vi "oscilloscope.vi"() -> ()   [LabVIEW 2017]
uses:
  <vilib>/DAQmx/read.llb/DAQmx Read (Analog Wfm 1Chan NSamp).vi
  <vilib>/DAQmx/create/channels.llb/DAQmx Create Channel (AI-Voltage-Basic).vi
  <vilib>/DAQmx/configure/timing.llb/DAQmx Timing (Sample Clock).vi
  <vilib>/DAQmx/miscellaneous.llb/DAQmx Fill In Error Info.vi
  <vilib>/Waveform/WDTOps.llb/WDT Get XY Value DBL.vi
panel:
  in  "physical channels":tag="cDAQ9185-1D03A69Mod1/ai14"
  out "Waveform Graph":waveform(dbl)(graph)
  out "Numeric":dbl
  in  "Stop Button":bool
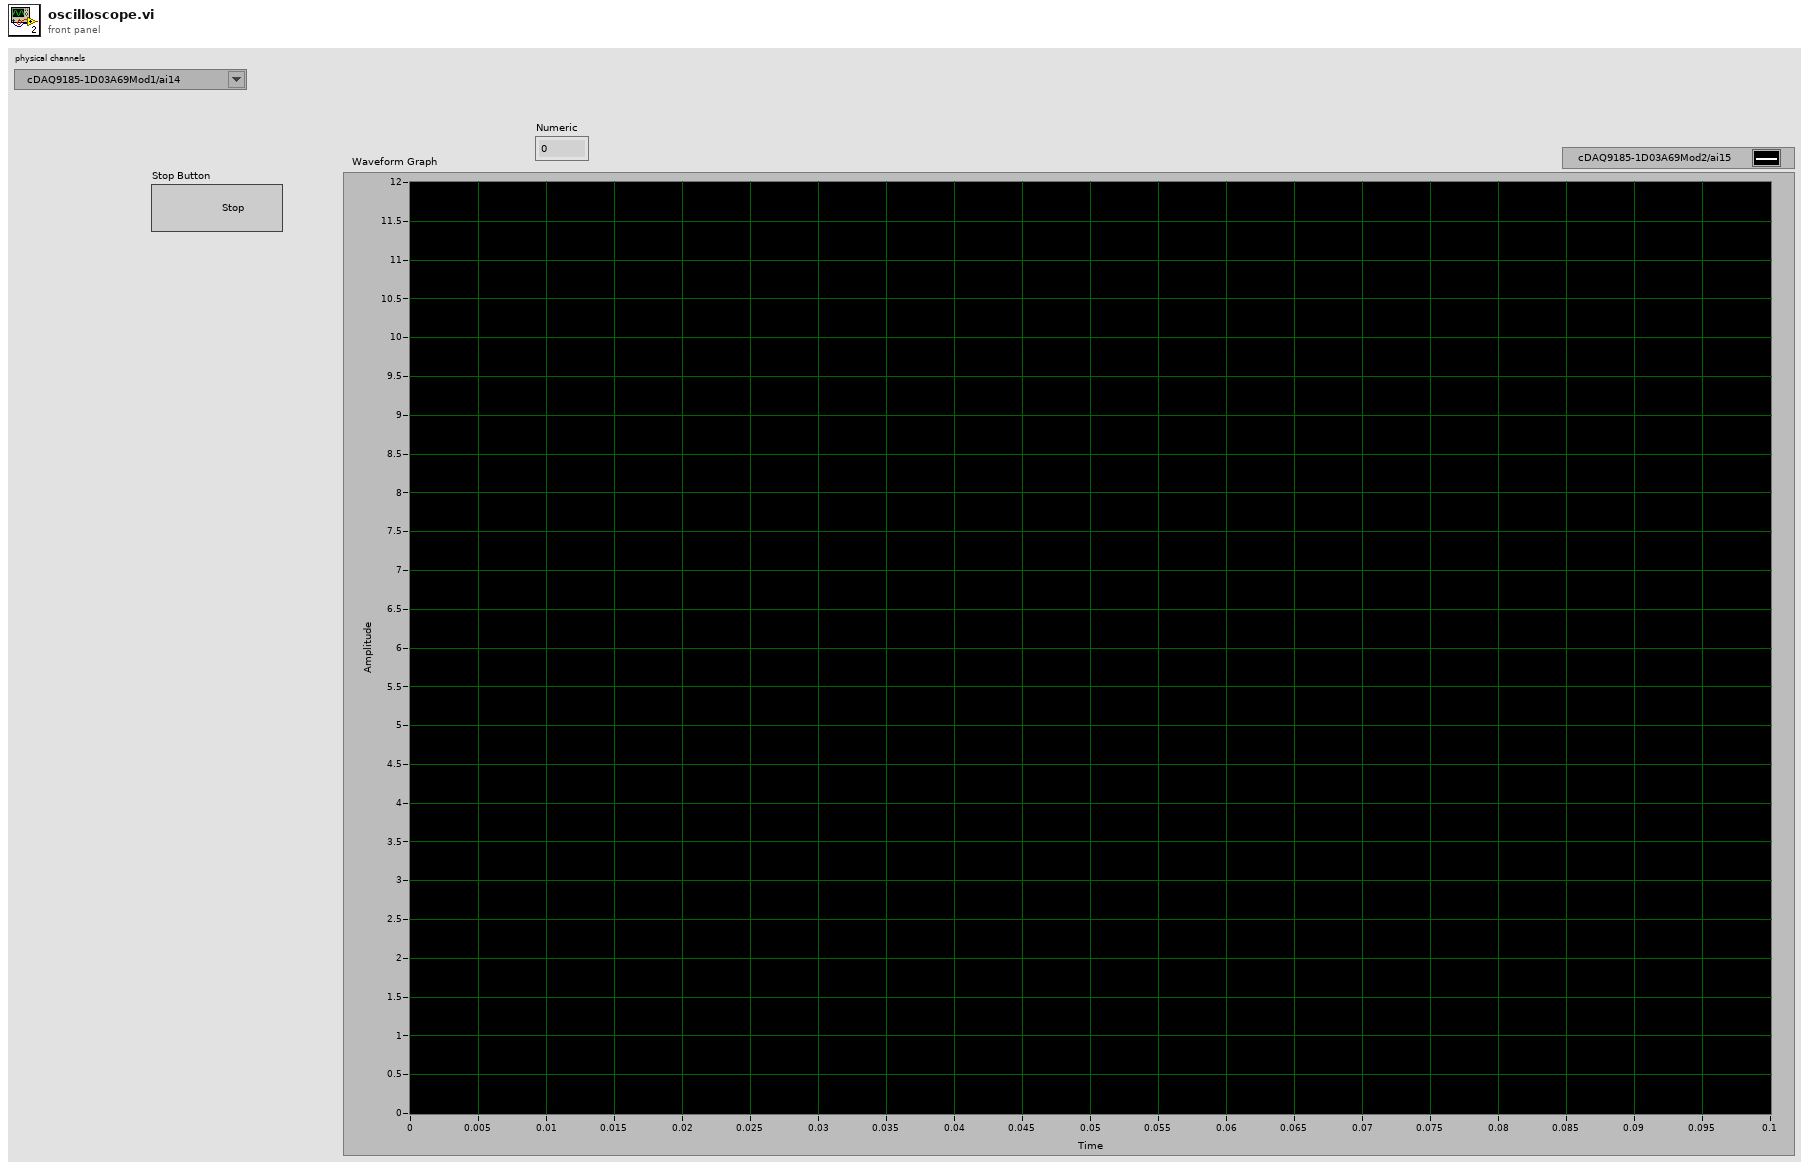
[diagram p1: front panel]
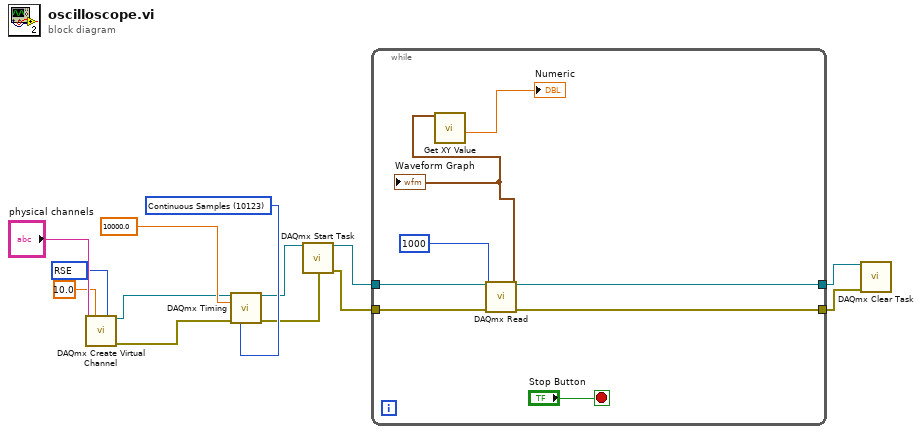
[diagram p0: block diagram]
diagram:
  w1 = 10083 items=["Default"=-1, "RSE"=10083, "NRSE"=10078, "Differential"=10106, "Pseudodifferential"=12529] ("input terminal configuration")
  w11 = 10123 items=["Finite Samples"=10178, "Continuous Samples"=10123, "Hardware Timed Single Point"=12522] ("sample mode")
  n1 = call-poly <vilib>:"DAQmx Create Virtual Channel.vi"("maximum value"=10.0, "input terminal configuration"=w1, "physical channels"="physical channels") -> ("task out"=w3:refnum<k21>, "error out"=w12:errorcluster)  [unwired: 11 in]
  n2 = call-poly <vilib>:"DAQmx Timing.vi"("task/channels in"=w3, "sample mode"=w11, "rate"=10000.0, "error in"=w12) -> ("task out"=w10:refnum<k21>, "error out"=w9:errorcluster)  [unwired: 10 in]
  n3 = call <vilib>:"DAQmx Start Task.vi"("task/channels in"=w10, "error in"=w9) -> ("task out"=w8:refnum<k21>, "error out"=w7:errorcluster)  [unwired: 12 in]
  n4 = while {
    tunnel: w8 -> [w21]
    tunnel: w7 -> [w20]
    tunnel: [w17] -> w5
    tunnel: [w16] -> w4
    stop <- "Stop Button" stop-if-true
    n5 = call-poly <vilib>:"DAQmx Read.vi"("task/channels in"=w21, "number of samples per channel"=1000, "error in"=w20) -> ("task out"=w17:refnum<k21>, "data"=w14:waveform(dbl), "error out"=w16:errorcluster)  [unwired: 10 in]
    "Waveform Graph" <- w14
    n6 = call-poly <vilib>:"Get XY Value.vi"("waveform in"=w14) -> ("Y value"=→"Numeric":dbl)  [unwired: 6 in, 4 out]
  }
  n7 = call <vilib>:"DAQmx Clear Task.vi"("task in"=w5, "error in"=w4) -> ()  [unwired: 13 in, 1 out]
